vi "loadDPScript.vi"(8 "error in (no error)":errorcluster, 11 "ExperimentRunner in":refnum<class "ExperimentRunner.lvclass">) -> (0 "error out":errorcluster, 3 "ExperimentRunner out":refnum<class "ExperimentRunner.lvclass">)   [LabVIEW 2011, in "Views.lvlib" / "ExperimentControl.lvlib" / "ExperimentRunner.lvclass"]
doc: "Loads a new path selected by user to the path array"
uses:
  ExperimentRunner.lvclass
  Tools/Filing/FileSystem/FileSystem.lvclass
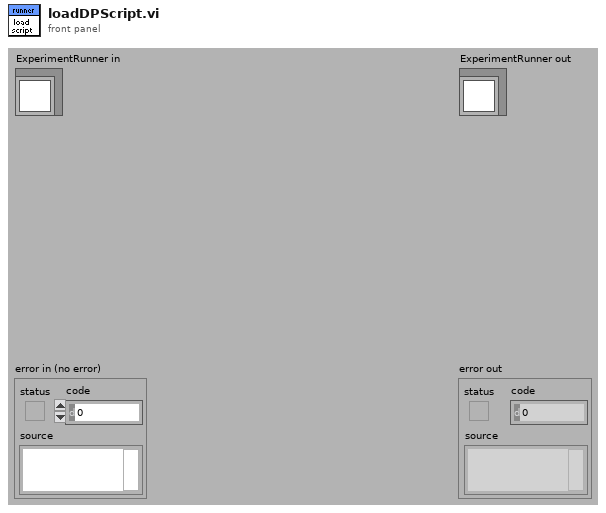
[diagram p1: front panel]
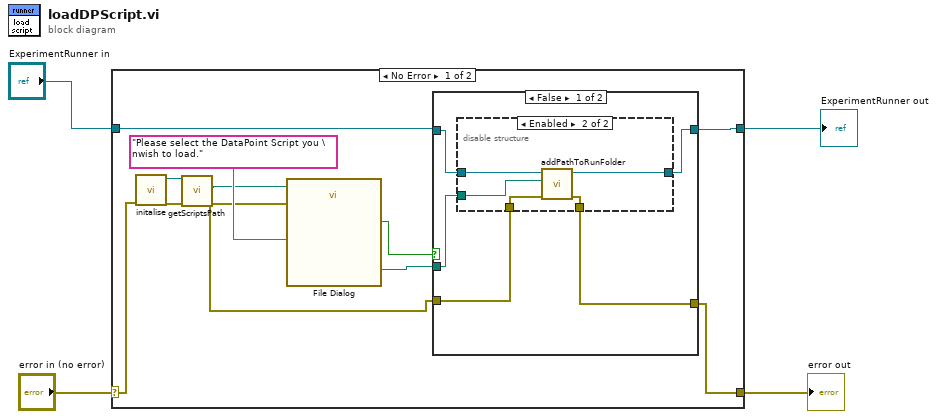
[diagram p0: block diagram]
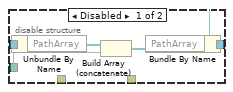
[diagram p2: hidden frame]
diagram:
  n1 = case shown="No Error" "error in (no error)" {
    selector: "error in (no error)" -> [w14 w34]
    tunnel: [w5 w34] -> w3
    tunnel: [w10 w33] -> w1
    tunnel: "ExperimentRunner in" -> [w12 w33]
    frame No Error {
      n2 = call "initalise.vi"("error in (no error)"=w14) -> ("error out"=w9:errorcluster, "FileSystem out"=w8:refnum<class "FileSystem.lvclass">)  [unwired: 9 in]
      n3 = call "getScriptsPath.vi"("error in (no error)"=w9, "FileSystem.lvclass in"=w8) -> ("error out"=w6:errorcluster, "Scripts"=w7:path)  [unwired: 7 in, 1 out]
      n4 = call "File Dialog"("start path"=w7, "prompt"="Please select the DataPoint Script you \nwish to load.", "error in"=w6) -> ("selected path"=w11:path, "cancelled"=w13:bool)  [unwired: 9 in, 2 out]
      n5 = case shown="False" w13 {
        tunnel: w12 -> [w19 w32]
        tunnel: w11 -> [w20 _]
        tunnel: [w18 w32] -> w10
        tunnel: w6 -> [w17 w31]
        tunnel: [w16 w31] -> w5
        frame False {
          n6 = disable-structure shown="Enabled" {
            disable-tunnel: w20 -> [w24 w29]
            disable-tunnel: w19 -> [w23 w30]
            disable-tunnel: [w22 w28] -> w18
            disable-tunnel: w17 -> [_ w27]
            disable-tunnel: [_ w26] -> w16
            frame Disabled {
              n7 = Unbundle By Name(w23) -> ("PathArray"=w25:path[])
              n8 = Build Array (concatenate)(w25, w24) -> (w21:path[])
              n9 = Bundle By Name(cluster=w23, "PathArray"=w21) -> (w22:refnum<class "ExperimentRunner.lvclass">)
            }
            frame Enabled {
              n10 = call "addPathToRunFolder.vi"("error in (no error)"=w27, "Path"=w29, "ExperimentRunner in"=w30) -> ("error out"=w26:errorcluster, "ExperimentRunner out"=w28:refnum<class "ExperimentRunner.lvclass">)  [unwired: 7 in]
            }
          }
        }
        frame True {
        }
      }
    }
    frame Error {
    }
  }
  "error out" <- w3
  "ExperimentRunner out" <- w1
